vi "Serialize.vi"(8 "error in (no error)":errorcluster, 11 "Board in":refnum<class "Board.lvclass">) -> (0 "error out":errorcluster, 2 "SerializedBoard":string, 3 "Board out":refnum<class "Board.lvclass">)   [LabVIEW 2015, in "TronviewGame.lvlib" / "Board.lvclass"]
uses:
  Board.lvclass
  Board.lvclass/Board.ctl
  Deserialize.vi
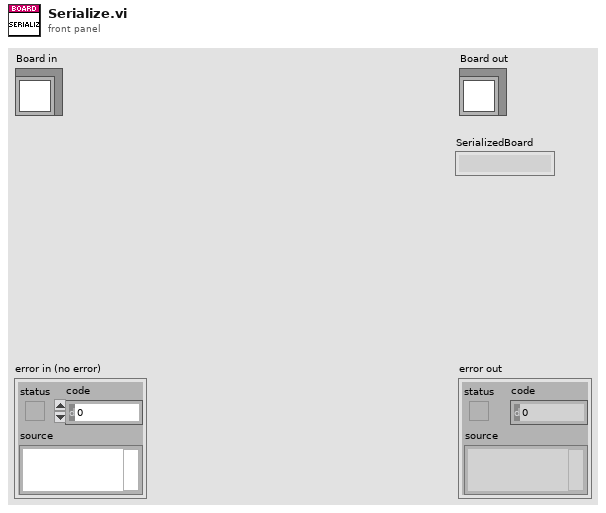
[diagram p1: front panel]
types:
  T1 = typedef "TronviewGame.lvlib/Board.lvclass/FieldState.ctl" = enum16{"Empty", "Blocked", "Player1Position", "Player2Postion", "Player1Marked", "Player2Marked"}
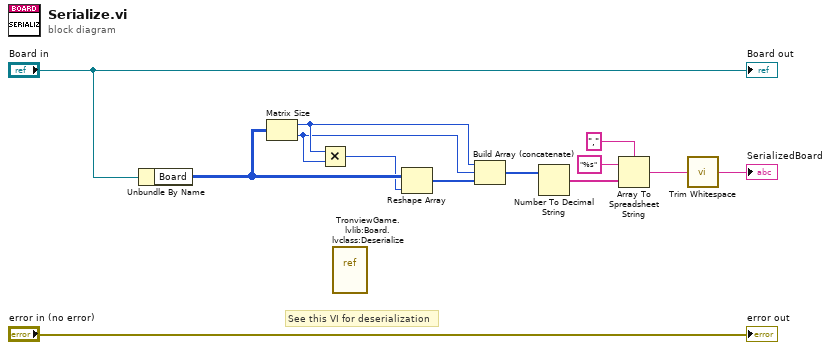
[diagram p0: block diagram]
diagram:
  # "See this VI for deserialization"
  n1 = Unbundle By Name("Board in") -> ("Board"=w11:T1[][])
  n2 = Matrix Size(0:w11) -> (1:w8:i32, 2:w7:i32)
  n3 = Multiply(x=w8, y=w7) -> (x*y=w9:i32)
  n4 = vi-ref "TronviewGame.lvlib:Board.lvclass:Deserialize.vi"() -> ()  [unwired: 1 out]
  n5 = Reshape Array(w11, w9) -> (w10:T1[])
  n6 = Build Array (concatenate)(w8, w7, w10) -> (w6:i32[])
  n7 = Number To Decimal String(number=w6) -> (decimal integer string=w5:string[])  [unwired: 1 in]
  n8 = Array To Spreadsheet String(delimiter (Tab)=",", array=w5, 3:"%s" ("format string")) -> (spreadsheet string=w2:string)
  n9 = call <vilib>:"Trim Whitespace.vi"("string"=w2) -> ("trimmed string"=→"SerializedBoard":string)  [unwired: 1 in]
  "error out" <- "error in (no error)"
  "Board out" <- "Board in"
